vi "DIO 4-bit.vi"(3 "DIO0 Refnum":refnum<k21>, 5 "DIO1 Refnum":refnum<k21>, 7 "DIO2 Refnum":refnum<k21>, 9 "DIR 3:0":fxp<+,4,4> format="%04b", 10 "OUT 3:0":fxp<+,4,4> format="%04b", 11 "DIO3 Refnum":refnum<k21>) -> (2 "IN 3:0":fxp<+,4,4> format="%04b")   [LabVIEW 2016]
doc: "This VI reads 4-bit data from or writes the data to the four specified FPGA I/O items according to the direction of the data flow (<b>DIR 3:0</b>).\nFor each bit of <b>DIR 3:0</b>:\n- DIR: 1 - Write data to the corresponding bit of <b>OUT 3:0</b>\n- DIR: 0 - Read data from the corresponding bit of <b>IN 3:0</b>"
panel:
  # "This VI reads 4-bit data from or writes the data to the four specified FPGA I/O items according to the direction of the data flow (DIR 3:0).\nFor each bit of DIR 3:0:\n- DIR: 1 - Write data to the corresponding bit of OUT 3:0\n- DIR: 0 - Read data from the corresponding bit of IN 3:0"
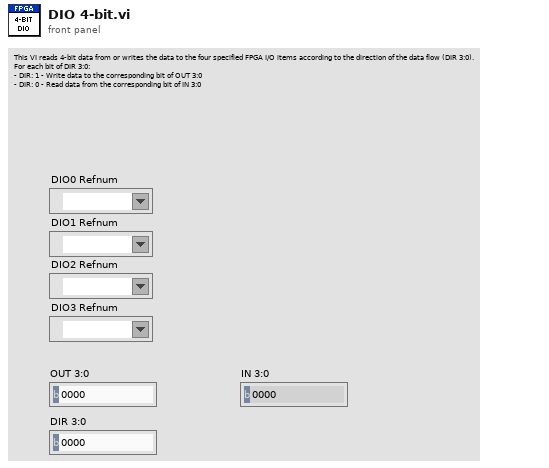
[diagram p1: front panel]
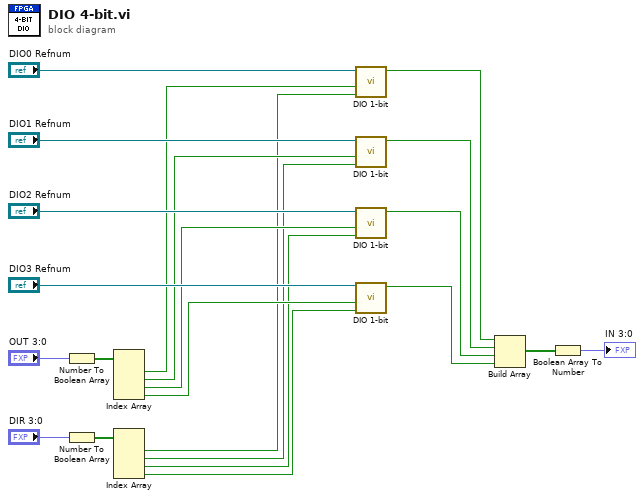
[diagram p0: block diagram]
diagram:
  n1 = Number To Boolean Array(number="OUT 3:0") -> (Boolean array=w16:bool[])
  n2 = Number To Boolean Array(number="DIR 3:0") -> (Boolean array=w11:bool[])
  n3 = Index Array(array=w16) -> (element #1=w15:bool, element #2=w14:bool, element #3=w13:bool, element #4=w12:bool)  [unwired: 4 in]
  n4 = Index Array(array=w11) -> (element #1=w10:bool, element #2=w9:bool, element #3=w8:bool, element #4=w7:bool)  [unwired: 4 in]
  n5 = call "DIO 1-bit.vi"("DIR"=w10, "OUT"=w15, "DIO Refnum"="DIO0 Refnum") -> ("IN"=w6:bool)  [unwired: 8 in]
  n6 = call "DIO 1-bit.vi"("DIR"=w9, "OUT"=w14, "DIO Refnum"="DIO1 Refnum") -> ("IN"=w5:bool)  [unwired: 8 in]
  n7 = call "DIO 1-bit.vi"("DIR"=w8, "OUT"=w13, "DIO Refnum"="DIO2 Refnum") -> ("IN"=w4:bool)  [unwired: 8 in]
  n8 = call "DIO 1-bit.vi"("DIR"=w7, "OUT"=w12, "DIO Refnum"="DIO3 Refnum") -> ("IN"=w3:bool)  [unwired: 8 in]
  n9 = Build Array(w6, w5, w4, w3) -> (w2:bool[])
  n10 = Boolean Array To Number(Boolean array=w2) -> (number=→"IN 3:0":fxp<+,4,4>)
